vi "append1DRow--string.vi"(6 "Style":refnum<class "Style.lvclass">, 8 "error in (no error)":errorcluster, 10 "Value":string[](array[string]), 11 "MS-Excel in":refnum<class "MS-Excel.lvclass">) -> (0 "error out":errorcluster, 3 "MS-Excel out":refnum<class "MS-Excel.lvclass">)   [LabVIEW 2020, in "LabVIEW NPOI.lvlib" / "MS-Excel.lvclass"]
uses:
  MS-Excel.lvclass
  Styles/Style/Style.lvclass
  MS-Excel.lvclass/MS-Excel.ctl
  D:/Benjamin/Documents/Perso/Code/WC/LVExcel/Resources/NPOI 2.1.1 dotnet2/NPOI.dll
  LVExcel/Resources/NPOI 2.1.1 dotnet2/NPOI.dll
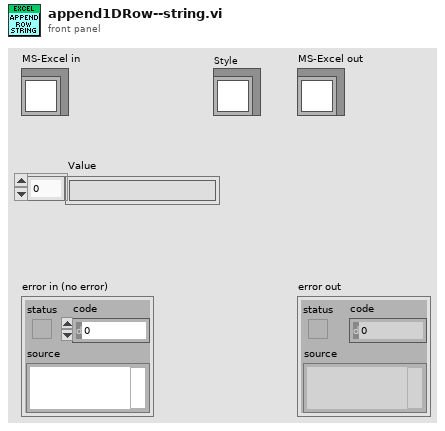
[diagram p1: front panel]
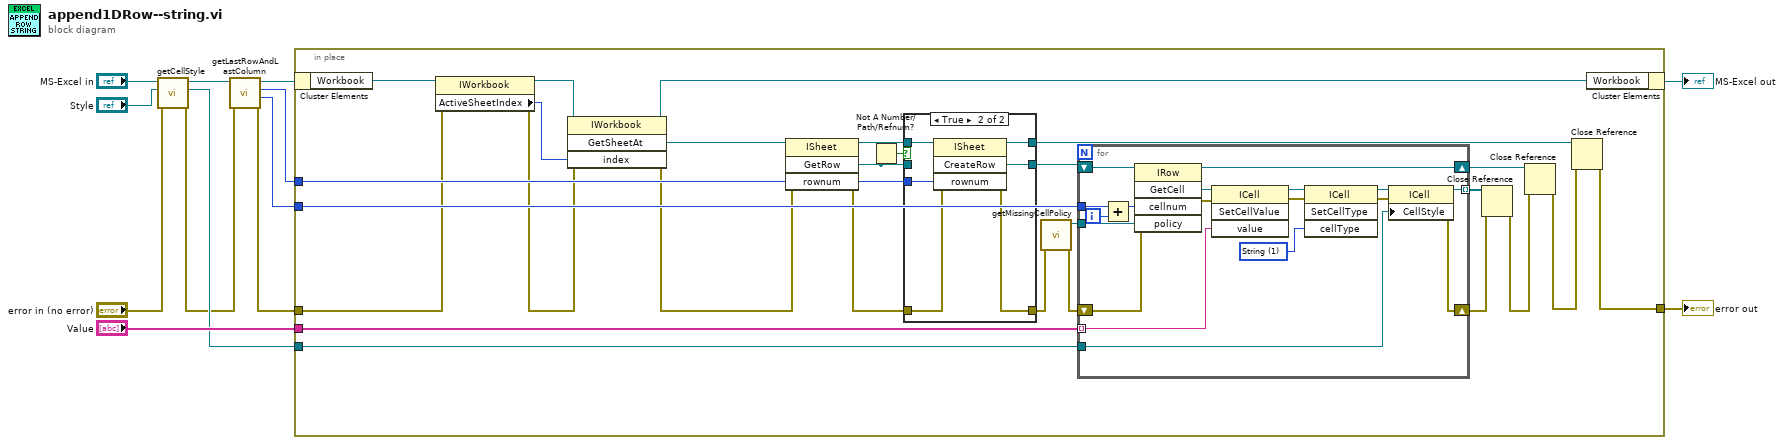
[diagram p0: block diagram]
diagram:
  n1 = call-dynamic "getCellStyle.vi"("error in (no error)"="error in (no error)", "Style"="Style", "MS-Excel in"="MS-Excel in") -> ("error out"=w1:errorcluster, "Cell Style"=w3:refnum<k24>, "MS-Excel out"=w5:refnum<class "MS-Excel.lvclass">)  [unwired: 6 in]
  n2 = call-dynamic "getLastRowAndLastColumn.vi"("error in (no error)"=w1, "MS-Excel in"=w5) -> ("error out"=w8:errorcluster, "Last Column"=w6:i32, "Last Row"=w7:i32, "MS-Excel out"=w9:refnum<class "MS-Excel.lvclass">)  [unwired: 6 in]
  n3 = in-place {
    in-place-border: w8 -> [w30]
    in-place-border: [w14] -> w12
    in-place-border: w7 -> [w40]
    in-place-border: w6 -> [w39]
    in-place-border: "Value" -> [w38]
    in-place-border: w3 -> [w27]
    n4 = in-place-cluster #1(w9) -> ("Workbook"=w28:refnum<k24>)
    n5 = property class="IWorkbook"(reference=w28, error in=w30) -> (reference out=w32:refnum<k24>, error out=w29:errorcluster, "ActiveSheetIndex"=w31:i32)
    n6 = invoke class="IWorkbook" method="GetSheetAt"(reference=w32, error in=w29, "index"=w31) -> (reference out=w34:refnum<k24>, error out=w33:errorcluster, "GetSheetAt"=w35:refnum<k24>)  [unwired: 1 in, 1 out]
    n7 = invoke class="ISheet" method="GetRow"(reference=w35, error in=w33, "rownum"=w40) -> (reference out=w24:refnum<k24>, error out=w23:errorcluster, "GetRow"=w25:refnum<k24>)  [unwired: 1 in, 1 out]
    n8 = Not A Number/Path/Refnum?(number/path/refnum=w25) -> (NaN/Path/Refnum?=w26:bool)
    n9 = case shown="True" w26 {
      tunnel: w25 -> [w60 _]
      tunnel: w24 -> [w59 w67]
      tunnel: w40 -> [_ w66]
      tunnel: w23 -> [w61 w62]
      tunnel: [w61 w64] -> w18
      tunnel: [w60 w65] -> w22
      tunnel: [w59 w63] -> w16
      frame False {
      }
      frame True {
        n10 = invoke class="ISheet" method="CreateRow"(reference=w67, error in=w62, "rownum"=w66) -> (reference out=w63:refnum<k24>, error out=w64:errorcluster, "CreateRow"=w65:refnum<k24>)  [unwired: 1 in, 1 out]
      }
    }
    n11 = call "getMissingCellPolicy.vi"("error in (no error)"=w18) -> ("error out"=w17:errorcluster, "CREATE_NULL_AS_BLANK"=w19:refnum<k24>)  [unwired: 9 in]
    n12 = for {
      shift-right: [w54] -> w37
      shift-left: w22 -> [w58]
      tunnel: w39 -> [w57]
      tunnel: w38 -> [w53] mode=indexing
      shift-right: [w41] -> w20
      shift-left: w17 -> [w52]
      tunnel: [w43] -> w21 mode=indexing
      tunnel: w19 -> [w46]
      tunnel: w27 -> [w44]
      i -> [w47]
      w48 = 1 items=["Numeric"=0, "String"=1, "Formula"=2, "Blank"=3, "Boolean"=4, "Error"=5, "Unknown"=-1] ("cellType")
      n13 = Add(x=w57, y=w47) -> (x+y=w56:i32)
      n14 = invoke class="IRow" method="GetCell"(reference=w58, error in=w52, "cellnum"=w56, "policy"=w46) -> (reference out=w54:refnum<k24>, error out=w51:errorcluster, "GetCell"=w55:refnum<k24>)  [unwired: 1 in, 2 out]
      n15 = invoke class="ICell" method="SetCellValue"(reference=w55, error in=w51, "value"=w53) -> (reference out=w50:refnum<k24>, error out=w49:errorcluster)  [unwired: 1 in, 2 out]
      n16 = invoke class="ICell" method="SetCellType"(reference=w50, error in=w49, "cellType"=w48) -> (reference out=w45:refnum<k24>, error out=w42:errorcluster)  [unwired: 1 in, 2 out]
      n17 = property class="ICell"(reference=w45, error in=w42, "CellStyle"=w44) -> (reference out=w43:refnum<k24>, error out=w41:errorcluster)
    }
    n18 = Close Reference(reference=w21, error in (no error)=w20) -> (error out=w36:errorcluster)
    n19 = Close Reference(reference=w37, error in (no error)=w36) -> (error out=w15:errorcluster)
    n20 = Close Reference(reference=w16, error in (no error)=w15) -> (error out=w14:errorcluster)
    n21 = in-place-cluster #1("Workbook"=w34) -> (→"MS-Excel out":refnum<class "MS-Excel.lvclass">)
  }
  "error out" <- w12
